vi "Read.vi"(7 "Slave Address":u8, 8 "Error In":errorcluster, 10 "Count":i32, 11 "I2C In":refnum<class "I2C.lvclass">) -> (0 "Error Out":errorcluster, 2 "Data":u8[](array[numeric]), 3 "I2C Out":refnum<class "I2C.lvclass">)   [LabVIEW 2020, in "lv_i2c_hal.lvlib" / "I2C.lvclass"]
uses:
  I2C.lvclass
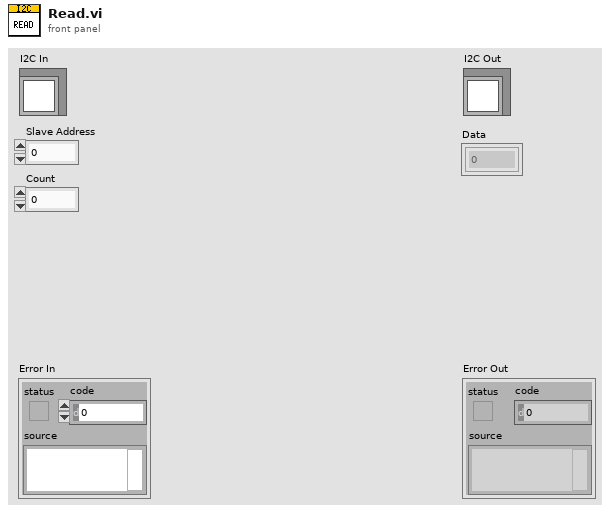
[diagram p1: front panel]
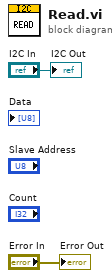
[diagram p0: block diagram]
diagram:
  "Error Out" <- "Error In"
  "I2C Out" <- "I2C In"
